vi "SetGrphScale.vi"(8 "error in (no error)":errorcluster caption="entrée d'erreur (pas d'erreur)", 10 "GraphIndex":i32, 11 "Interface en entrée":refnum<class "Interface.lvclass"> caption="Interface Class in") -> (0 "error out":errorcluster caption="sortie d'erreur", 3 "Interface en sortie":refnum<class "Interface.lvclass"> caption="DNL_LabVIEW Object out")   [LabVIEW 2019, in "Interface.lvclass"]
uses:
  Interface.lvclass
  Interface.lvclass/Interface.ctl
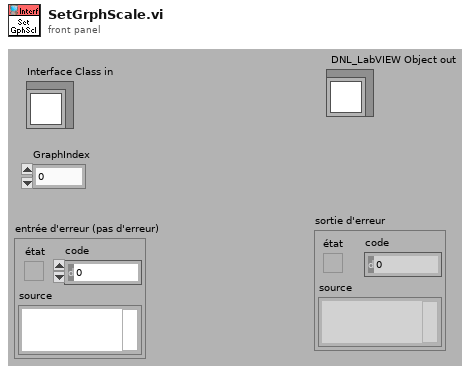
[diagram p1: front panel]
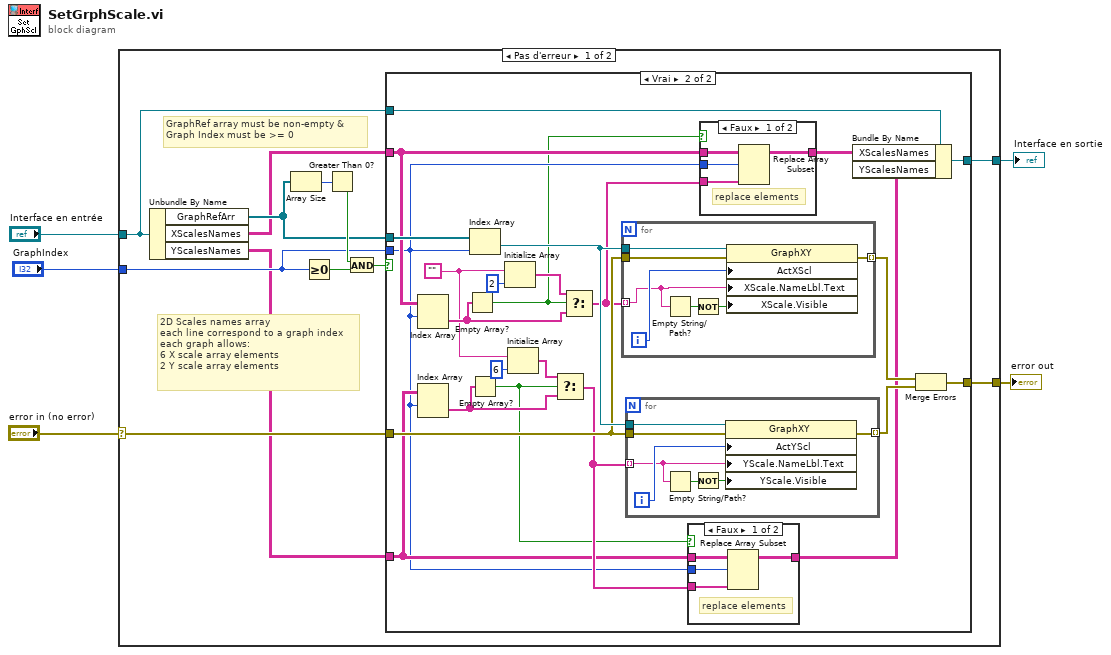
[diagram p0: block diagram]
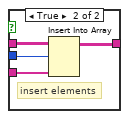
[diagram p3: hidden frame]
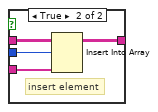
[diagram p4: hidden frame]
diagram:
  n1 = case shown="Pas d'erreur" "error in (no error)" {
    selector: "error in (no error)" -> [w10 w74]
    tunnel: "GraphIndex" -> [w12 _]
    tunnel: [w11 w74] -> w4
    tunnel: "Interface en entrée" -> [w7 w75]
    tunnel: [w8 w75] -> w2
    frame No Error {
      # "GraphRef array must be non-empty &\nGraph Index must be >= 0"
      # "2D Scales names array\neach line correspond to a graph index\neach graph allows:\n6 X scale array elements\n2 Y scale array elements"
      n2 = Unbundle By Name(w7) -> ("GraphRefArr"=w14:refnum<vi>[], "XScalesNames"=w9:string[][], "YScalesNames"=w6:string[][])
      n3 = Array Size(array=w14) -> (size(s)=w17:i32)
      n4 = Greater Or Equal To 0?(x=w12) -> (x >= 0?=w15:bool)
      n5 = Greater Than 0?(x=w17) -> (x > 0?=w16:bool)
      n6 = And(x=w16, y=w15) -> (x .and. y?=w13:bool)
      n7 = case shown="Vrai" w13 {
        tunnel: w14 -> [_ w43]
        tunnel: w12 -> [_ w24]
        tunnel: [w19 w39] -> w11
        tunnel: w10 -> [w19 w38]
        tunnel: w9 -> [_ w28]
        tunnel: [w18 w32] -> w8
        tunnel: w7 -> [w18 w33]
        tunnel: w6 -> [_ w26]
        frame False {
        }
        frame True {
          w22 = ""
          n8 = Index Array(array=w28, index (row)=w24) -> (element=w27:string[])  [unwired: 1 in]
          n9 = Index Array(array=w26, index (row)=w24) -> (element=w25:string[])  [unwired: 1 in]
          n10 = Empty Array?(array=w27) -> (empty?=w21:bool)
          n11 = Index Array(array=w43, index=w24) -> (element=w42:refnum<vi>)
          n12 = Empty Array?(array=w25) -> (empty?=w20:bool)
          n13 = Initialize Array(w22, 2 ("taille de la dimension")) -> (w35:string[])
          n14 = Initialize Array(w22, 6 ("taille de la dimension")) -> (w36:string[])
          n15 = Select(t=w36, s=w20, f=w25) -> (s? t:f=w29:string[])
          n16 = Select(t=w35, s=w21, f=w27) -> (s? t:f=w34:string[])
          n17 = for {
            tunnel: w42 -> [w73]
            tunnel: [w71] -> w41 mode=indexing
            tunnel: w38 -> [w70]
            tunnel: w34 -> [w67] mode=indexing
            i -> [w72]
            n18 = Empty String/Path?(string/path=w67) -> (empty?=w68:bool)
            n19 = Not(x=w68) -> (.not. x?=w69:bool)
            n20 = property class="GraphXY"(reference=w73, error in=w70, "ActXScl"=w72, "XScale.NameLbl.Text"=w67, "XScale.Visible"=w69) -> (error out=w71:errorcluster)  [unwired: 1 out]
          }
          n21 = for {
            tunnel: w42 -> [w66]
            tunnel: w29 -> [w60] mode=indexing
            tunnel: [w63] -> w40 mode=indexing
            tunnel: w38 -> [w62]
            i -> [w65]
            n22 = Empty String/Path?(string/path=w60) -> (empty?=w61:bool)
            n23 = Not(x=w61) -> (.not. x?=w64:bool)
            n24 = property class="GraphXY"(reference=w66, error in=w62, "ActYScl"=w65, "YScale.NameLbl.Text"=w60, "YScale.Visible"=w64) -> (error out=w63:errorcluster)  [unwired: 1 out]
          }
          n25 = case shown="Faux" w20 {
            tunnel: [w47 w50] -> w30
            tunnel: w29 -> [w46 w49]
            tunnel: w26 -> [w45 w51]
            tunnel: w24 -> [w44 w48]
            frame False {
              # "replace elements"
              n26 = Replace Array Subset(array=w45, new element=w46, index (row)=w44) -> (w47:string[][])  [unwired: 1 in]
            }
            frame True {
              # "insert elements"
              n27 = Insert Into Array(array=w51, index (row)=w48, new element=w49) -> (w50:string[][])  [unwired: 1 in]
            }
          }
          n28 = case shown="Faux" w21 {
            tunnel: w34 -> [w55 w57]
            tunnel: [w54 w58] -> w31
            tunnel: w28 -> [w53 w59]
            tunnel: w24 -> [w52 w56]
            frame False {
              # "replace elements"
              n29 = Replace Array Subset(array=w53, new element=w55, index (row)=w52) -> (w54:string[][])  [unwired: 1 in]
            }
            frame True {
              # "insert element"
              n30 = Insert Into Array(array=w59, index (row)=w56, new element=w57) -> (w58:string[][])  [unwired: 1 in]
            }
          }
          n31 = Bundle By Name(cluster=w33, "XScalesNames"=w31, "YScalesNames"=w30) -> (w32:refnum<class "Interface.lvclass">)
          n32 = Merge Errors(w41, w40) -> (w39:errorcluster)
        }
      }
    }
    frame Error {
    }
  }
  "Interface en sortie" <- w2
  "error out" <- w4
